vi "Create All Message Queues.vi"(8 "error in (no error)":errorcluster, 11 "This VI":refnum<vi>) -> (0 "error out":errorcluster, 3 "Message Queues out":T1)   [LabVIEW 2024, in "Keyence_VS150.lvlib" / "Message Queue.lvlib"]
doc: "This VI creates and initializes all the message queues for your application. If your application requires more than one message queue, right-click the \"Message Queues\" constant above and select Open Type Def. Add the new Message Queue(s) to the type definition, then initialize them in this VI."
uses:
  Message Queue.lvlib
  All Message Queues.ctl
  Enqueue Message (Single).vi
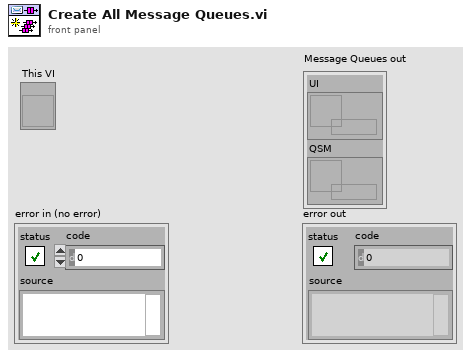
[diagram p1: front panel]
types:
  T1 = typedef "Keyence_VS150.lvlib/Message Queue.lvlib/All Message Queues.ctl" = cluster{"UI":refnum<queue>, "QSM":refnum<queue>}
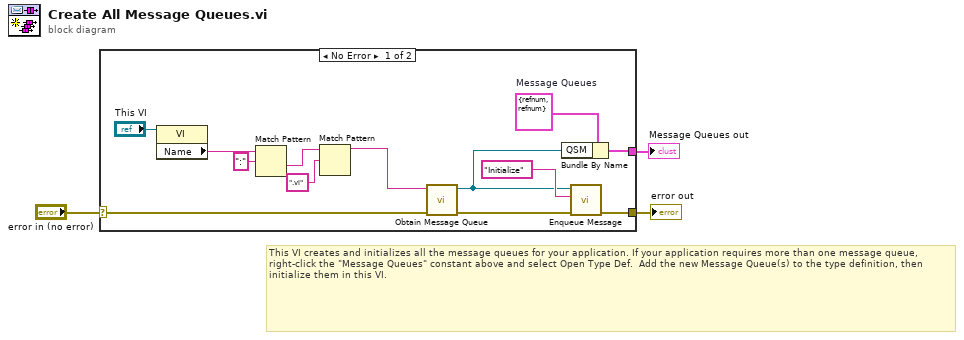
[diagram p0: block diagram]
diagram:
  # "This VI creates and initializes all the message queues for your application. If your application requires more than one message queue, right-click the \"Message Queues\" constant above and select Open Type Def.  Add the new Message Queue(s) to the type definition, then initialize them in this VI."
  n1 = case shown="No Error" "error in (no error)" {
    selector: "error in (no error)" -> [w13 w17]
    tunnel: [w16 w17] -> w3
    tunnel: [w14 _] -> w2
    frame No Error {
      w15 = T1 {"UI"=refnum, "QSM"=refnum}  # Message Queues
      n2 = property class="VI"(reference="This VI") -> ("Name"=w4:string)  [unwired: 1 in, 2 out]
      n3 = Match Pattern(string=w4, regular expression=":") -> (after substring=w7:string)  [unwired: 1 in, 3 out]
      n4 = Match Pattern(string=w7, regular expression=".vi") -> (before substring=w5:string)  [unwired: 1 in, 3 out]
      n5 = call "Obtain Message Queue.vi"("error in (no error)"=w13, "Queue"=w5) -> ("error out"=w12:errorcluster, "Message Queue"=w10:refnum<queue>)  [unwired: 8 in]
      n6 = Bundle By Name(cluster=w15, "QSM"=w10) -> (w14:T1)
      n7 = call-poly "Enqueue Message.vi"("error in (no error)"=w12, "Message"="Initialize", "Message Queue"=w10) -> ("error out"=w16:errorcluster)  [unwired: 7 in, 1 out]
    }
    frame Error {
    }
  }
  "Message Queues out" <- w2
  "error out" <- w3
